vi "Periodic Tasks.vi"(8 "error in":errorcluster) -> ()   [LabVIEW 2015]
doc: "This VI runs in parallel to other tasks. It can contain as many user-defined periodic loops as you need. These can carry out PID or other sorts of timed response."
uses:
  NavX Library/navX Library v2/TypeDefs/Z900_navX_DeviceTypeDef.ctl
  NavX Library/navX Library v2/TypeDefs/Z900_navX_ProtocolTypeDef.ctl
  NavX Library/navX Library v2/TypeDefs/Z900_navX_NotifyPacketTypeDef.ctl
  NavX Library/navX Library v2/TypeDefs/Z900_navX_ActionTypeDef.ctl
  <vilib>/Rock Robotics/WPI/Utilities/WPI_GetSetVariantRefNum.vi
  Robot Global Data.vi
  <vilib>/Rock Robotics/Network Tables/SD Write Number.vi
  NavX Library/navX Library v2/navX Library v2.lvlib
panel:
  in  "navX Device":T1={"Interface"={"Protocol"=enum."SPI", "Update Rate (4Hz-60Hz)"=50, "navX Open TypeDef"=variant(cluster{"DevStatus":errorcluster, "Handle":i32, "Controller":enum16{"Controller 1"}, "SPI Bus":enum16{"SPI On-Board, CS0", "SPI On-Board, CS1", "SPI On-Board, CS2", "SPI On-Board, CS3", "SPI MXP", "Invalid"}} {"DevStatus"={"status"=FALSE, "code"=0, "source"=""}, "Handle"=0, "Controller"=enum."Controller 1", "SPI Bus"=enum."SPI On-Board, CS0"})}, "Notify Packet"=refnum, "Loop VI Refnum"=refnum, "Ready to Close Occurrence Refnum"=refnum} {"Interface"."Update Rate (4Hz-60Hz)" min=4 max=60 step=1}
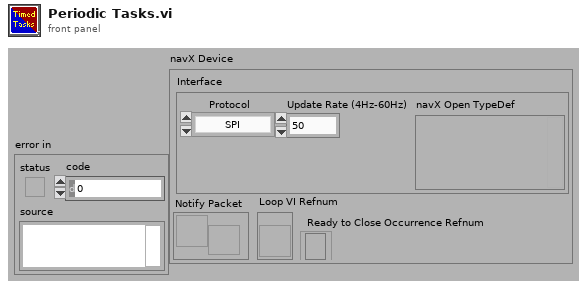
[diagram p1: front panel]
types:
  T1 = typedef "navX Library v2.lvlib/Z900_navX_DeviceTypeDef.ctl" = cluster{"Interface":cluster{"Protocol":T2, "Update Rate (4Hz-60Hz)":u8, "navX Open TypeDef":variant}, "Notify Packet":refnum<notifier>, "Loop VI Refnum":refnum<vi>, "Ready to Close Occurrence Refnum":refnum<k4>}
  T2 = typedef "navX Library v2.lvlib/Z900_navX_ProtocolTypeDef.ctl" = enum16{"SERIAL", "I2C", "SPI"}
  T3 = typedef "WPI_JoystickDevRef.ctl" = cluster{"Device":T4}
  T4 = typedef "WPI_JoystickDeviceEnum.ctl" = enum16{"USB 0", "USB 1", "USB 2", "USB 3", "USB 4", "USB 5"}
  T5 = cluster{"Axes[0]":dbl, "Axes[1]":dbl, "Axes[2]":dbl, "Axes[3]":dbl, "Axes[4]":dbl, "Axes[5]":dbl, "Axes[6]":dbl, "Axes[7]":dbl, "Axes[8]":dbl}
  T6 = cluster{"Buttons[0]":bool, "Buttons[1]":bool, "Buttons[2]":bool, "Buttons[3]":bool, "Buttons[4]":bool, "Buttons[5]":bool, "Buttons[6]":bool, "Buttons[7]":bool, "Buttons[8]":bool}
  T7 = cluster{"LinearAcceleration X":dbl, "LinearAcceleration Y":dbl, "LinearAcceleration Z":dbl}
  T8 = cluster{"Velocity X":dbl, "Velocity Y":dbl, "Velocity Z":dbl, "Displacement X":dbl, "Displacement Y":dbl, "Displacement Z":dbl}
  T9 = cluster{"Yaw":dbl, "Roll":dbl, "Pitch":dbl, "Heading":dbl, "Fused Heading":dbl}
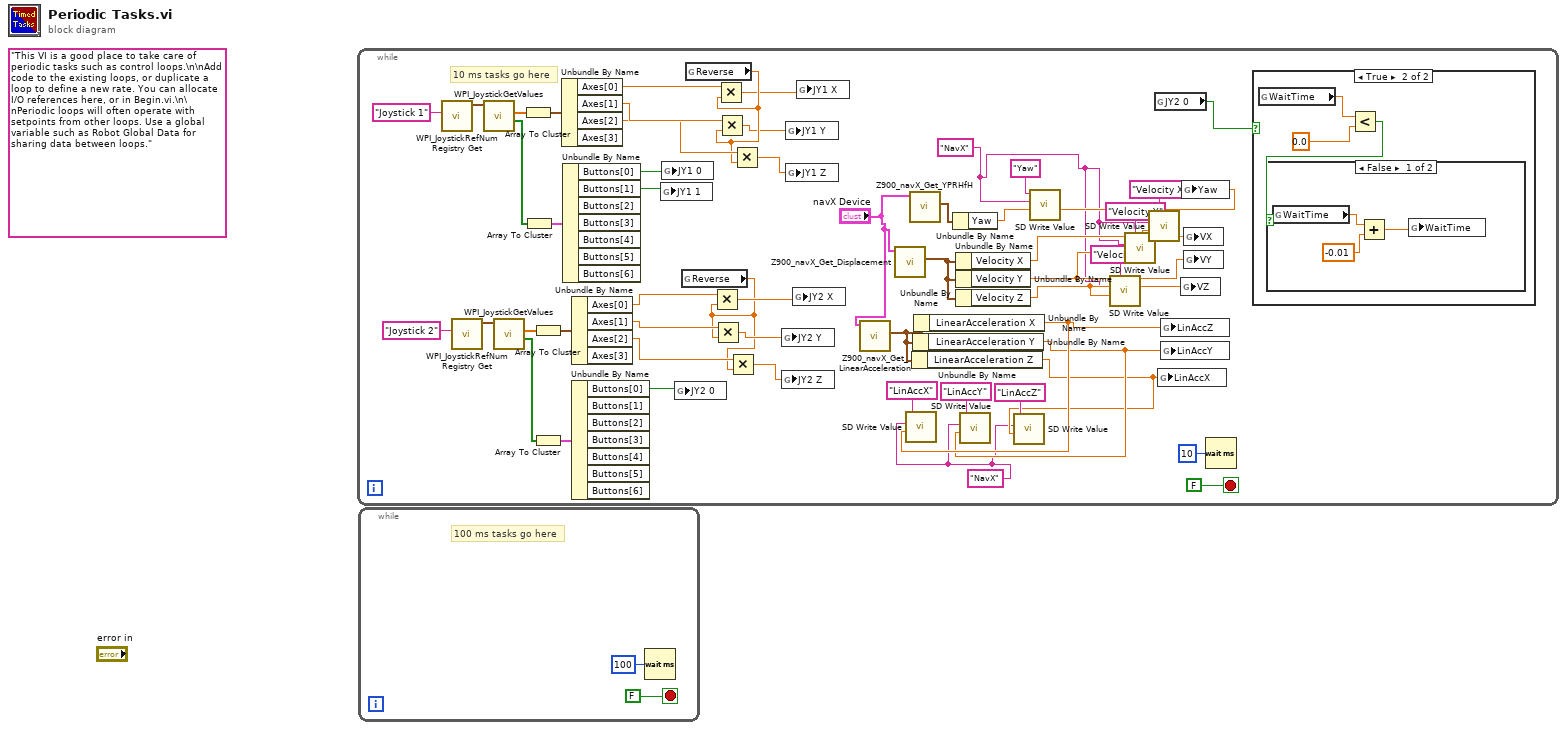
[diagram p0: block diagram]
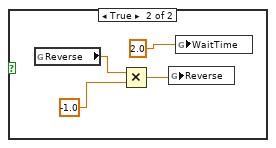
[diagram p3: hidden frame]
diagram:
  (unwired) "This VI is a good place to take care of periodic tasks such as control loops.\n\nAdd code to the existing loops, or duplicate a loop to define a new rate. You can allocate I/O references here, or in Begin.vi.\n\nPeriodic loops will often operate with setpoints from other loops. Use a global variable such as Robot Global Data for sharing data between loops."
  n1 = while {
    stop <- FALSE stop-if-true
    w6 = "NavX"
    w13 = "NavX"
    # "10 ms tasks go here"
    n2 = call <vilib>:"WPI_JoystickRefNum Registry Get.vi"("refnum name"="Joystick 1") -> ("JoystickDevRef"=w49:T3)  [unwired: 1 in, 9 out]
    n3 = call <vilib>:"WPI_JoystickRefNum Registry Get.vi"("refnum name"="Joystick 2") -> ("JoystickDevRef"=w43:T3)  [unwired: 1 in, 9 out]
    n4 = call <vilib>:"WPI_JoystickGetValues.vi"("JoystickDevRef"=w49) -> ("Buttons"=w47:bool[], "Axes"=w46:dbl[])  [unwired: 6 in, 3 out]
    n5 = call <vilib>:"WPI_JoystickGetValues.vi"("JoystickDevRef"=w43) -> ("Buttons"=w41:bool[], "Axes"=w40:dbl[])  [unwired: 6 in, 3 out]
    n6 = Array To Cluster(array=w46) -> (cluster=w48:T5)
    n7 = Array To Cluster(array=w47) -> (cluster=w45:T6)
    n8 = Array To Cluster(array=w40) -> (cluster=w42:T5)
    n9 = Array To Cluster(array=w41) -> (cluster=w39:T6)
    n10 = Unbundle By Name(w48) -> ("Axes[0]"=w35:dbl, "Axes[1]"=w34:dbl, "Axes[2]"=w33:dbl)  [unwired: 1 out]
    n11 = Unbundle By Name(w45) -> ("Buttons[0]"=w38:bool, "Buttons[1]"=w37:bool)  [unwired: 5 out]
    n12 = Unbundle By Name(w42) -> ("Axes[0]"=w25:dbl, "Axes[1]"=w24:dbl, "Axes[2]"=w23:dbl)  [unwired: 1 out]
    n13 = Unbundle By Name(w39) -> ("Buttons[0]"=w36:bool)  [unwired: 6 out]
    n14 = global write "Robot Global Data.vi" "JY1 1"(w37) -> ()
    n15 = global write "Robot Global Data.vi" "JY1 0"(w38) -> ()
    n16 = global write "Robot Global Data.vi" "JY2 0"(w36) -> ()
    n17 = global read "Robot Global Data.vi" "Reverse"() -> (w22:dbl)
    n18 = global read "Robot Global Data.vi" "Reverse"() -> (w32:dbl)
    n19 = Multiply(x=w25, y=w22) -> (x*y=w28:dbl)
    n20 = Multiply(x=w24, y=w22) -> (x*y=w27:dbl)
    n21 = Multiply(x=w35, y=w32) -> (x*y=w31:dbl)
    n22 = Multiply(x=w34, y=w32) -> (x*y=w30:dbl)
    n23 = Multiply(x=w23, y=w22) -> (x*y=w26:dbl)
    n24 = Multiply(x=w33, y=w32) -> (x*y=w29:dbl)
    n25 = global write "Robot Global Data.vi" "JY2 Y"(w27) -> ()
    n26 = global write "Robot Global Data.vi" "JY2 Z"(w26) -> ()
    n27 = global write "Robot Global Data.vi" "JY1 Y"(w30) -> ()
    n28 = global write "Robot Global Data.vi" "JY1 Z"(w29) -> ()
    n29 = global write "Robot Global Data.vi" "JY2 X"(w28) -> ()
    n30 = global write "Robot Global Data.vi" "JY1 X"(w31) -> ()
    n31 = call "Z900_navX_Get_LinearAcceleration.vi"("navX Device"="navX Device") -> ("Linear Acceleration"=w4:T7)  [unwired: 7 in, 3 out]
    n32 = call "Z900_navX_Get_Displacement.vi"("navX Device"="navX Device") -> ("Displacement"=w2:T8)  [unwired: 7 in, 3 out]
    n33 = call "Z900_navX_Get_YPRHfH.vi"("navX Device"="navX Device") -> ("YRPHfH"=w3:T9)  [unwired: 7 in, 3 out]
    n34 = Unbundle By Name(w4) -> ("LinearAcceleration Z"=w7:dbl)
    n35 = Unbundle By Name(w4) -> ("LinearAcceleration Y"=w8:dbl)
    n36 = Unbundle By Name(w4) -> ("LinearAcceleration X"=w9:dbl)
    n37 = call-poly <vilib>:"SD Write Value.vi"("Numeric"=w9, "Table Prefix"=w6, "Name"="LinAccX") -> ()  [unwired: 7 in, 2 out]
    n38 = Unbundle By Name(w3) -> ("Yaw"=w20:dbl)
    n39 = Unbundle By Name(w2) -> ("Velocity X"=w18:dbl)
    n40 = Unbundle By Name(w2) -> ("Velocity Y"=w16:dbl)
    n41 = Unbundle By Name(w2) -> ("Velocity Z"=w14:dbl)
    n42 = call-poly <vilib>:"SD Write Value.vi"("Numeric"=w8, "Table Prefix"=w6, "Name"="LinAccY") -> ()  [unwired: 7 in, 2 out]
    n43 = call-poly <vilib>:"SD Write Value.vi"("Numeric"=w7, "Table Prefix"=w6, "Name"="LinAccZ") -> ()  [unwired: 7 in, 2 out]
    n44 = call-poly <vilib>:"SD Write Value.vi"("Numeric"=w20, "Table Prefix"=w13, "Name"="Yaw") -> ()  [unwired: 7 in, 2 out]
    n45 = call-poly <vilib>:"SD Write Value.vi"("Numeric"=w14, "Table Prefix"=w13, "Name"="Velocity Z") -> ()  [unwired: 7 in, 2 out]
    n46 = call-poly <vilib>:"SD Write Value.vi"("Numeric"=w16, "Table Prefix"=w13, "Name"="Velocity Y") -> ()  [unwired: 7 in, 2 out]
    n47 = call-poly <vilib>:"SD Write Value.vi"("Numeric"=w18, "Table Prefix"=w13, "Name"="Velocity X") -> ()  [unwired: 7 in, 2 out]
    n48 = global read "Robot Global Data.vi" "JY2 0"() -> (w5:bool)
    n49 = global write "Robot Global Data.vi" "LinAccX"(w7) -> ()
    n50 = global write "Robot Global Data.vi" "LinAccZ"(w9) -> ()
    n51 = global write "Robot Global Data.vi" "LinAccY"(w8) -> ()
    n52 = global write "Robot Global Data.vi" "VZ"(w14) -> ()
    n53 = global write "Robot Global Data.vi" "Yaw"(w20) -> ()
    n54 = global write "Robot Global Data.vi" "VX"(w18) -> ()
    n55 = global write "Robot Global Data.vi" "VY"(w16) -> ()
    n56 = Wait (ms)(milliseconds to wait=u32 10) -> ()  [unwired: 1 out]
    n57 = case shown="True" w5 {
      frame False {
      }
      frame True {
        n58 = global read "Robot Global Data.vi" "WaitTime"() -> (w55:dbl)
        n59 = Less?(x=w55, y=0.0) -> (x < y?=w53:bool)
        n60 = case shown="False" w53 {
          frame False {
            n61 = global read "Robot Global Data.vi" "WaitTime"() -> (w58:dbl)
            n62 = Add(x=w58, y=-0.01) -> (x+y=w56:dbl)
            n63 = global write "Robot Global Data.vi" "WaitTime"(w56) -> ()
          }
          frame True {
            n64 = global read "Robot Global Data.vi" "Reverse"() -> (w61:dbl)
            n65 = Multiply(x=w61, y=-1.0) -> (x*y=w60:dbl)
            n66 = global write "Robot Global Data.vi" "Reverse"(w60) -> ()
            n67 = global write "Robot Global Data.vi" "WaitTime"(2.0) -> ()
          }
        }
      }
    }
  }
  n68 = while {
    stop <- FALSE stop-if-true
    # "100 ms tasks go here"
    n69 = Wait (ms)(milliseconds to wait=u32 100) -> ()  [unwired: 1 out]
  }
